vi "图像对称、曲面操作3.vi"() -> ()   [LabVIEW 2018]
uses:
  <vilib>/vision/NI_Vision_Development_Module.lvlib
panel:
  out "Image 4":T1(plugin-control)
  out "Image 3":T1(plugin-control)
  out "error out":errorcluster
  out "Image 2":T1(plugin-control)
  out "Image":T1(plugin-control)
  in  "路径":path
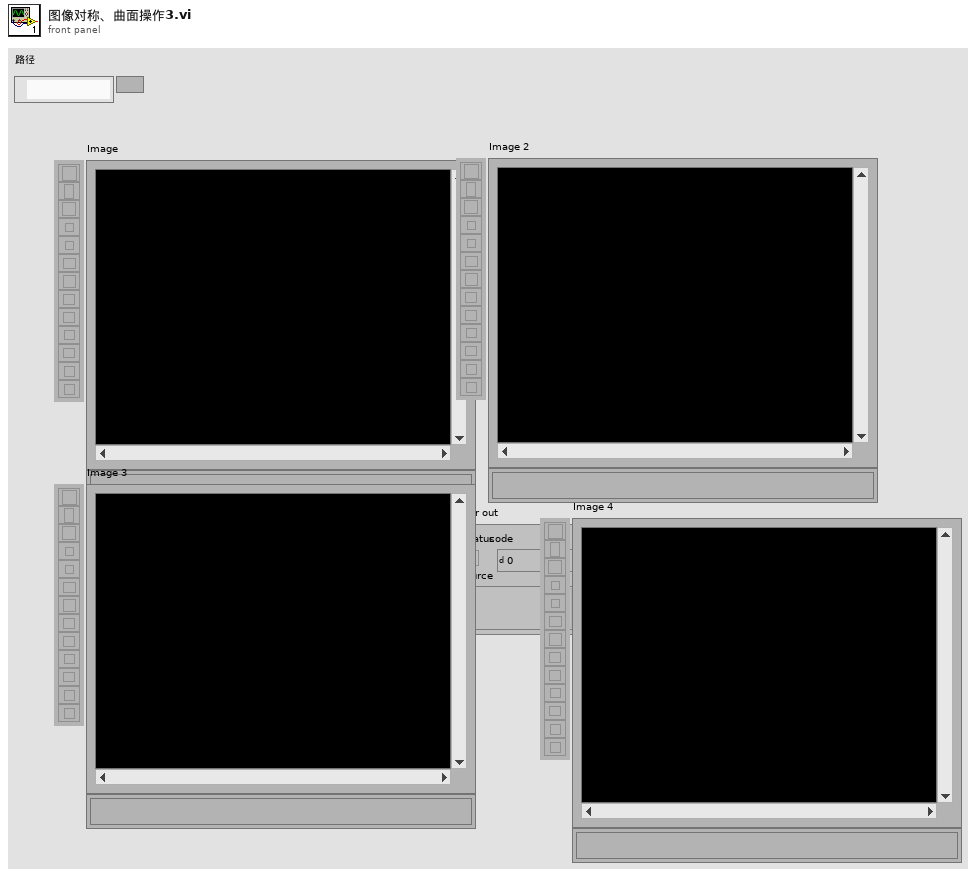
[diagram p1: front panel]
types:
  T1 = typedef "IMAQ Image.ctl" = refnum<image>
  T2 = typedef "IMAQ Circle" = cluster{"Center X":i32, "Center Y":i32, "Inner Radius":i32, "Outer Radius":i32, "Start Angle":dbl, "End Angle":dbl}
  T3 = typedef "ROI Descriptor" = cluster{"Global Rectangle":i32[], "Contours":cluster{"ID":enum32{"External", "Internal"}, "Type":u32, "Coordinates":i32[]}[]}
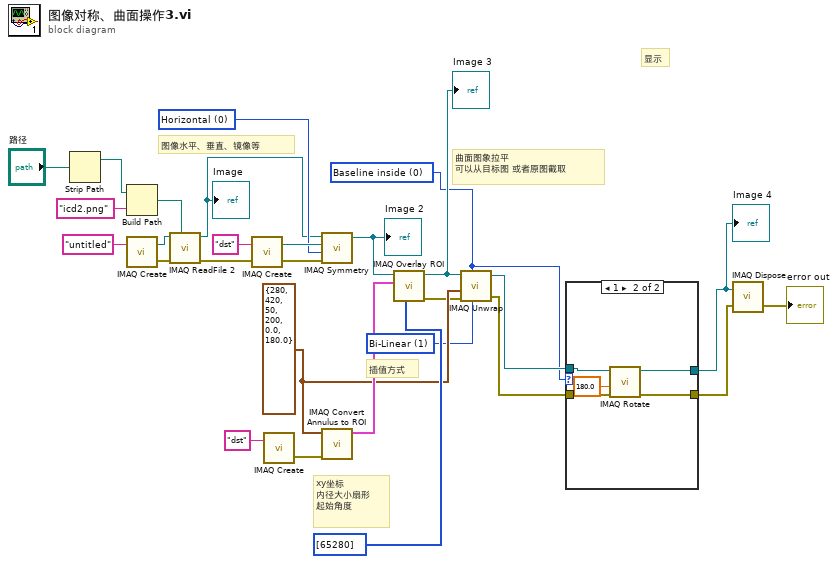
[diagram p0: block diagram]
diagram:
  w4 = u32 0 items=["Baseline inside", "Baseline outside"] ("Orientation")
  w6 = u32 1 items=["Zero Order", "Bi-Linear", "Quadratic", "Cubic Spline"] ("Interpolation Type")
  w9 = T2 {"Center X"=280, "Center Y"=420, "Inner Radius"=50, "Outer Radius"=200, "Start Angle"=0.0, "End Angle"=180.0} ("Annulus")
  w18 = u32 0 items=["Horizontal", "Vertical", "Central", "1st Diagonal", "2nd Diagonal"] ("Type of Symmetry")
  # "插值方式"
  # "显示"
  # "xy坐标\n内径大小扇形\n起始角度"
  # "曲面图象拉平\n可以从目标图 或者原图截取"
  # "图像水平、垂直、镜像等"
  n1 = Strip Path(path="路径") -> (stripped path=w27:path)  [unwired: 1 out]
  n2 = Build Path(base path=w27, name or relative path="icd2.png" ("名称或相对路径")) -> (appended path=w16:path)
  n3 = call "IMAQ Create"("Image Name"="untitled") -> ("New Image"=w25:T1, "error out"=w24:errorcluster)  [unwired: 4 in]
  n4 = call "IMAQ ReadFile 2"("File Path"=w16, "error in (no error)"=w24, "Image"=w25) -> ("error out"=w22:errorcluster, "Image Out"=w17:T1)  [unwired: 4 in, 3 out]
  "Image" <- w17
  n5 = call "IMAQ Create"("Image Name"="dst", "error in (no error)"=w22) -> ("New Image"=w20:T1, "error out"=w19:errorcluster)  [unwired: 3 in]
  n6 = call "IMAQ Create"("Image Name"="dst") -> ("error out"=w13:errorcluster)  [unwired: 4 in, 1 out]
  n7 = call "IMAQ Symmetry"("error in (no error)"=w19, "Type of Symmetry"=w18, "Image Dst"=w20, "Image Src"=w17) -> ("Image Dst Out"=w12:T1)  [unwired: 1 in, 1 out]
  "Image 2" <- w12
  n8 = call "IMAQ Convert Annulus to ROI"("error in (no error)"=w13, "Annulus"=w9) -> ("ROI Descriptor"=w11:T3)  [unwired: 7 in, 1 out]
  n9 = call "IMAQ Overlay ROI"("Colors (Green)"=u32[] [65280], "ROI Descriptor"=w11, "Image"=w12) -> ("error out"=w7:errorcluster, "Image Out"=w8:T1)  [unwired: 7 in]
  "Image 3" <- w8
  n10 = call "IMAQ Unwrap"("Image Src"=w8, "Orientation"=w4, "Annulus"=w9, "Interpolation Type"=w6, "error in (no error)"=w7) -> ("Image Dst Out"=w5:T1, "error out"=w3:errorcluster)  [unwired: 2 in]
  n11 = case shown="1" w4 {
    tunnel: w5 -> [w30 w35]
    tunnel: w3 -> [w29 w34]
    tunnel: [w30 w33] -> w1
    tunnel: [w29 w32] -> w2
    frame 0, Default {
    }
    frame 1 {
      n12 = call "IMAQ Rotate"("error in (no error)"=w34, "Angle (degrees)"=sgl 180.0, "Image Src"=w35) -> ("error out"=w32:errorcluster, "Image Dst Out"=w33:T1)  [unwired: 7 in]
    }
  }
  "Image 4" <- w1
  n13 = call "IMAQ Dispose"("Image"=w1, "error in (no error)"=w2) -> ("error out"=→"error out":errorcluster)  [unwired: 4 in]
